vi "CoordinateTransform.vi"(0 "error in (no error)":errorcluster, 2 "input coordiantes":cluster{"x":dbl, "y":dbl}={"x"=0.0, "y"=100.0}, 3 "Conversion Matrix":dbl[][](array[numeric])=[[1.0, 0.0, 0.0], [0.0, 0.9999999999999996, 0.0]], 4 "back":bool) -> (1 "error out":errorcluster, 5 "output coordiantes":cluster{"x":dbl, "y":dbl}={"x"=1.9429894176211716e-14, "y"=99.99999999999996})   [LabVIEW 2011]
uses:
  <vilib>/Analysis/baseanly.llb/A x Vector.vi
  <vilib>/Analysis/NI_AALBase.lvlib
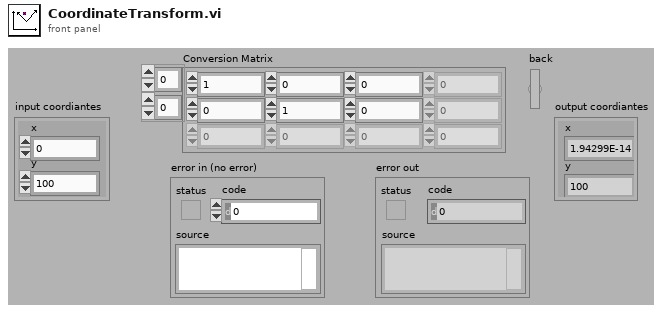
[diagram p1: front panel]
types:
  T1 = cluster{"A x Vector[0]":dbl, "A x Vector[1]":dbl}
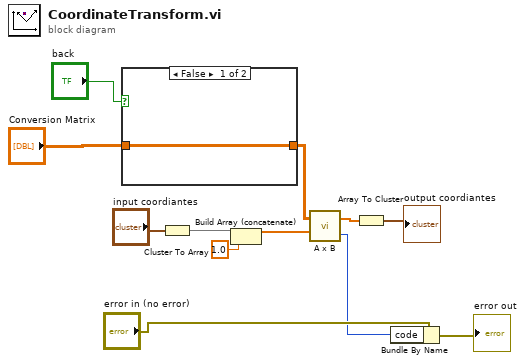
[diagram p0: block diagram]
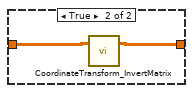
[diagram p2: hidden frame]
diagram:
  n1 = case shown="False" "back" {
    tunnel: "Conversion Matrix" -> [w13 w15]
    tunnel: [w13 w14] -> w2
    frame False {
    }
    frame True {
      n2 = call "CoordinateTransform_InvertMatrix.vi"("Conversion Matrix"=w15) -> ("invers Conversion Matrix"=w14:dbl[][])  [unwired: 1 in, 1 out]
    }
  }
  n3 = Cluster To Array(cluster="input coordiantes") -> (array=w11:dbl[])
  n4 = Build Array (concatenate)(w11, 1.0) -> (w9:dbl[])
  n5 = call-poly <vilib>:"A x B.vi"("Vector"=w9, "A"=w2) -> ("error"=w4:i32, "A x Vector"=w8:dbl[])
  n6 = Array To Cluster(array=w8) -> (cluster=→"output coordiantes":T1)
  n7 = Bundle By Name(cluster="error in (no error)", "code"=w4) -> (→"error out":errorcluster)
